vi "Get CurWeek(0).vi"(8 "error in (no error)":errorcluster, 11 "Admin_Actor in":refnum<class "Admin_Actor.lvclass">) -> (0 "error out":errorcluster, 2 "CurWeek(0)":i32, 3 "Admin_Actor out":refnum<class "Admin_Actor.lvclass">)   [LabVIEW 2015, in "Admin_Actor.lvlib" / "Admin_Actor.lvclass"]
uses:
  Admin_Actor.lvclass
  Admin_Actor.lvclass/Admin_Actor.ctl
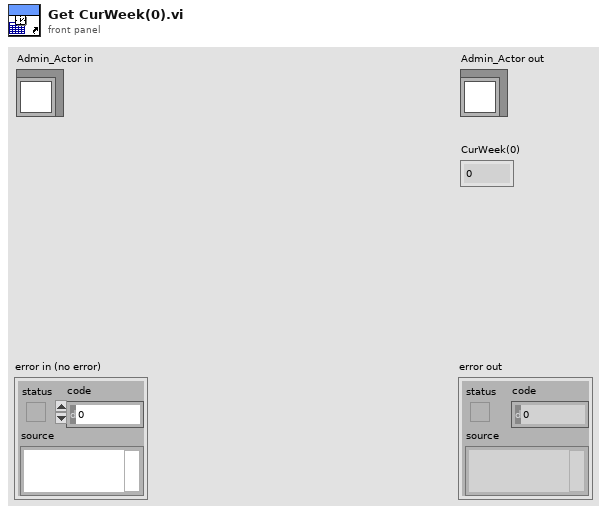
[diagram p1: front panel]
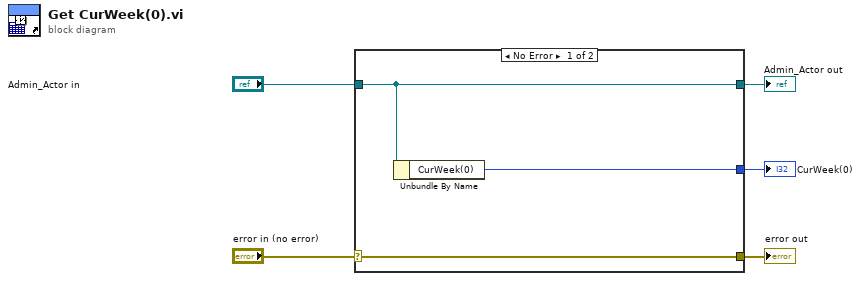
[diagram p0: block diagram]
diagram:
  n1 = case shown="No Error" "error in (no error)" {
    selector: "error in (no error)" -> [w8 w9]
    tunnel: [w8 w9] -> w4
    tunnel: [w7 w10] -> w2
    tunnel: "Admin_Actor in" -> [w7 w10]
    tunnel: [w6 _] -> w1
    frame No Error {
      n2 = Unbundle By Name(w7) -> ("CurWeek(0)"=w6:i32)
    }
    frame Error {
    }
  }
  "error out" <- w4
  "Admin_Actor out" <- w2
  "CurWeek(0)" <- w1
